vi "test_conv2.vi"() -> ()   [LabVIEW 2018]
uses:
  <vilib>/Analysis/1siggen.llb/Ramp Pattern by Samples.vi
  <vilib>/addons/Modulation/Digital/General/MT Generate Bits (Galois, PN Order).vi
  <vilib>/Analysis/baseanly.llb/Mean (DBL).vi
  <vilib>/addons/Modulation/Analog/support/mod_Set Error Source.vi
  <vilib>/addons/Modulation/Digital/Support/Common/Validators/mod_Generate Bits Validate.vi
  <vilib>/addons/Modulation/Digital/Support/Common/Validators/mod_AWGN Validate.vi
  <vilib>/addons/Modulation/Digital/Impairments/subVIs/mod_createSeeds.vi
  <vilib>/addons/Modulation/Digital/Support/Common/Validators/mod_Validate Samples Per Symbol.vi
  <vilib>/addons/Modulation/Analog/support/Validators/mod_Validate Complex Waveform.vi
  <vilib>/addons/Modulation/Analog/support/Validators/mod_WFErrorHandler.vi
  <vilib>/addons/Modulation/Digital/Support/Common/Validators/mod_Generate Filter Coefficients Validate.vi
  <vilib>/addons/Modulation/Digital/General/subVIs/mod_Generate Filter Coefficients.vi
  <vilib>/addons/Modulation/Digital/General/MT Generate PSK System Parameters(M).vi
  <vilib>/addons/Modulation/Digital/General/subVIs/mod_Generate Bits PN Sequence.vi
  <vilib>/Analysis/1siggen.llb/Gaussian White Noise (obs 90).vi
  <vilib>/addons/Modulation/Digital/General/MT Apply Matched Filter (Generic).vi
  <vilib>/addons/Modulation/Digital/General/MT Map PSK Symbols to Bits.vi
  <vilib>/addons/Modulation/Digital/Channel Coding/MT Convolutional Decoder (Viterbi Hard Decision, Rate).vi
  <vilib>/addons/Modulation/Digital/Demodulation/MT Calculate BER After Trigger (PN Sequence).vi
  <vilib>/addons/Modulation/niDMT.lvlib
  <vilib>/Analysis/NI_AALBase.lvlib
panel:
  out "size(s) 4":i32
  out "bruité":cdb[](array[numeric])
  out "built-in decoder":i8[](array[numeric])
  in  "Traceback Depth (D)":i32=20
  in  "Constraint Length (K)":i32=3
  in  "Rate (k/n)":enum16{"1/2", "1/3", "1/4", "2/3", "3/4"}(ring)
  in  "PN Sequence Order":i32=19
  in  "Seed In":i32=-1
  out "BER vs Eb/N0 (dB)\n[AWGN channel]":cluster{"Ramp Pattern":dbl[], dbl[]}(graph)
  in  "Trials per Eb/N0 Sample":i32=1
  in  "Start Eb/N0 (dB)":dbl=5.0 format="%0.2f"
  in  "End Eb/N0 (dB)":dbl=10.0 format="%0.2f"
  in  "Eb/N0 Samples":i32=6
  out "Progress in current trial":i32(slide) scale=0.0..100.0
  out "Accumulated BER (coding)":dbl format="%.4p"
  out "IQ Constellation":T1(graph)
  out "Y":cdb[](array[numeric])
  out "out_perso":i8[](array[numeric])
  out "size(s)":i32
  out "size(s) 2":i32
  out "message":i8[](array[numeric])
  out "size(s) 3":i32
  out "mess_codé":i8[](array[numeric])
  out "built-in CAN":i8[](array[numeric])
  out "Current trial":i32
  out "Current Eb/N0":dbl
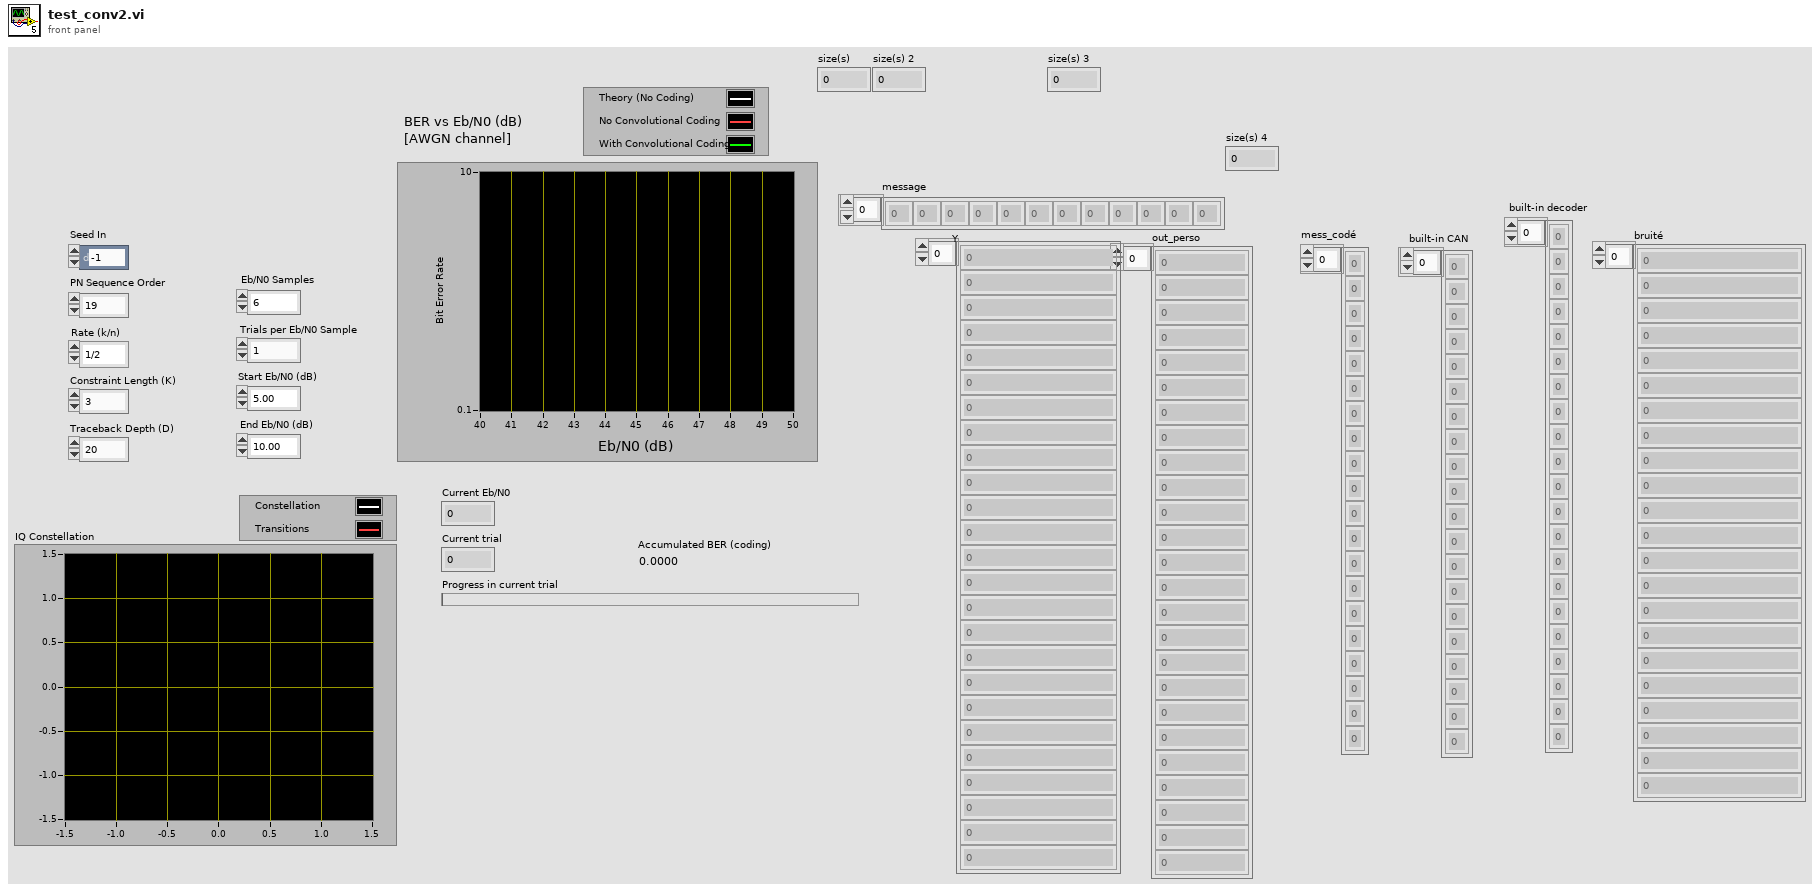
[diagram p1: front panel]
types:
  T1 = cluster{"Decimated Array":dbl[], "Decimated Array":dbl[]}[]
  T2 = enum16{"none", "Raised Cosine", "Root Raised Cos", "Gaussian"}
  T3 = cluster{"samples per symbol (16)":i32, "symbol map":cdb[], "differential PSK":enum16{"disable", "enable"}, "PSK type":u16}
  T4 = typedef "niAMT.lvlib/Complex Data Waveform.ctl" = cluster{"t0":dbl, "dt":dbl, "Y":cdb[]}
  T5 = cluster{"constellation":dbl[], "oversampled data":dbl[]}[]
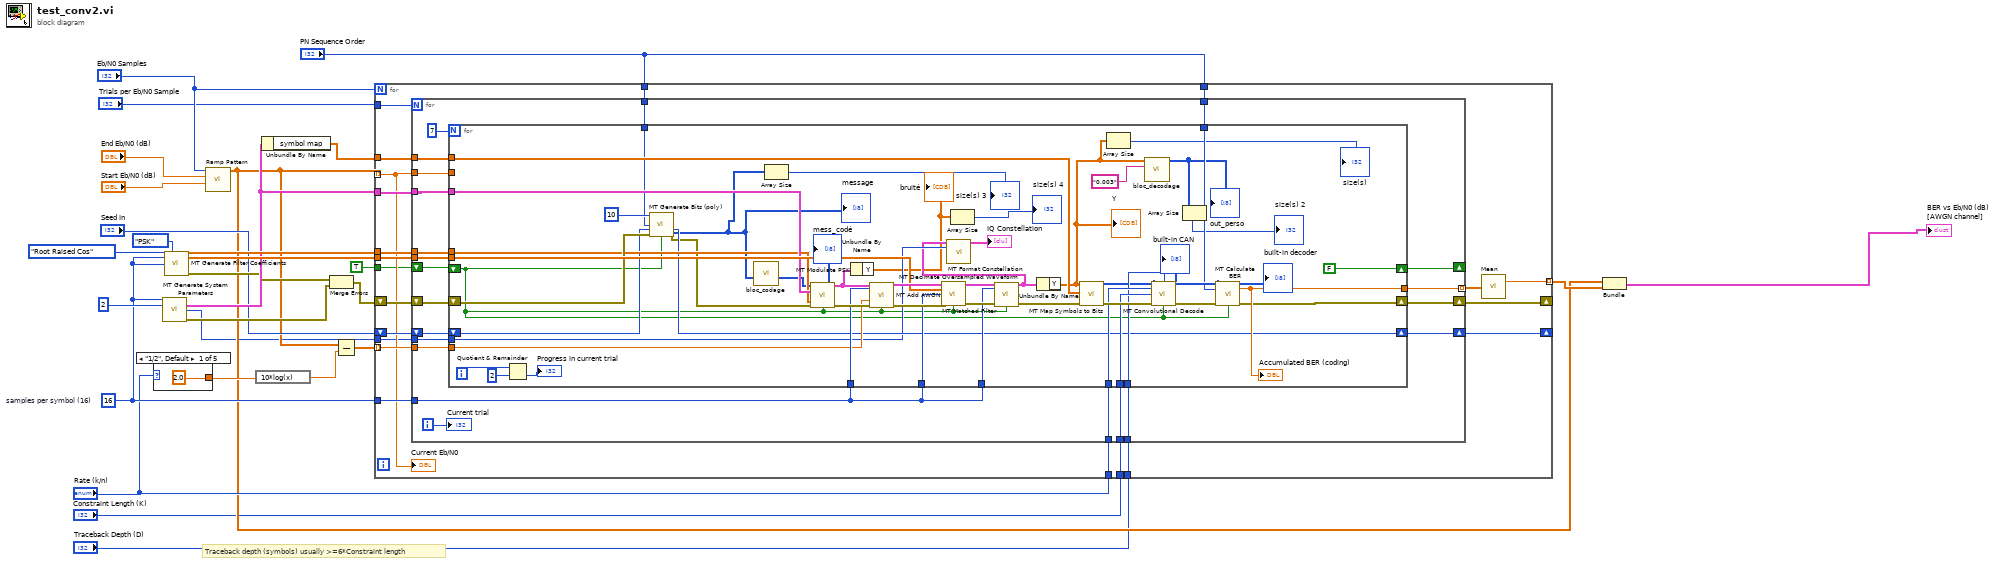
[diagram p0: block diagram]
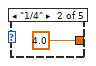
[diagram p2: hidden frame]
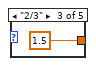
[diagram p3: hidden frame]
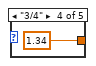
[diagram p4: hidden frame]
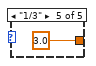
[diagram p5: hidden frame]
diagram:
  w21 = 16  # samples per symbol (16)
  # "Traceback depth (symbols) usually >=6*Constraint length"
  n1 = case shown="\"1/2\", Default" "Rate (k/n)" {
    tunnel: [2.0 4.0 1.5 1.34 3.0] -> w8
    frame "1/2", Default {
    }
    frame "1/4" {
    }
    frame "2/3" {
    }
    frame "3/4" {
    }
    frame "1/3" {
    }
  }
  n2 = call-poly <vilib>:"MT Generate System Parameters.vi"("samples per symbol (16)"=w21, "M-PSK (4)"=2) -> ("PSK system parameters"=w20:T3, "bits per symbol"=w2:i32, "error out"=w15:errorcluster)  [unwired: 11 in]
  n3 = call <vilib>:"MT Generate Filter Coefficients.vi"("pulse shaping filter (none)"=T2."Root Raised Cos", "modulation type"=enum16{"FSK", "PSK", "QAM", "MSK", "PAM", "ASK"}."PSK", "pulse shaping samples per symbol (16)"=w21, "matched samples per symbol (16)"=w21) -> ("pulse shaping filter coefficients"=w26:dbl[], "matched filter coefficients"=w22:dbl[], "error out"=w16:errorcluster)  [unwired: 9 in]
  n4 = call-poly <vilib>:"Ramp Pattern.vi"("start"="Start Eb/N0 (dB)", "end"="End Eb/N0 (dB)", "samples"="Eb/N0 Samples") -> ("Ramp Pattern"=w6:dbl[])  [unwired: 7 in, 1 out]
  n5 = expression code="10*log(x)"(w8) -> (w7:dbl)
  n6 = Unbundle By Name(w20) -> ("symbol map"=w19:cdb[])
  n7 = Merge Errors(w16, w15) -> (w14:errorcluster)
  n8 = Subtract(x=w6, y=w7) -> (x-y=w13:dbl[])
  n9 = for {
    N: "Eb/N0 Samples" -> [_]
    tunnel: w26 -> [w54]
    tunnel: w6 -> [w36] mode=indexing
    tunnel: w22 -> [w52]
    tunnel: w21 -> [w51]
    tunnel: w19 -> [w50]
    tunnel: "Rate (k/n)" -> [w49]
    tunnel: "Constraint Length (K)" -> [w48]
    tunnel: "Traceback Depth (D)" -> [w47]
    tunnel: "Trials per Eb/N0 Sample" -> [w46]
    tunnel: [w44] -> w10 mode=indexing
    tunnel: w20 -> [w53]
    shift-right: [w43] -> _
    shift-left: w14 -> [w42]
    tunnel: w13 -> [w41] mode=indexing
    shift-right: [w39] -> _
    shift-left: "Seed In" -> [w40]
    tunnel: "PN Sequence Order" -> [w38]
    tunnel: "PN Sequence Order" -> [w37]
    tunnel: TRUE ("reset? (T)") -> [w35]
    tunnel: w2 -> [w34]
    n10 = for {
      N: w46 -> [_]
      tunnel: w54 -> [w76]
      tunnel: w36 -> [w74]
      tunnel: w52 -> [w73]
      tunnel: w51 -> [w72]
      tunnel: w50 -> [w71]
      tunnel: w49 -> [w70]
      tunnel: w48 -> [w69]
      tunnel: w47 -> [w68]
      tunnel: [w66] -> w45 mode=indexing
      tunnel: w53 -> [w75]
      shift-right: [w64] -> w43
      shift-left: w42 -> [w63]
      tunnel: w41 -> [w62]
      shift-right: [w60] -> w39
      shift-left: w40 -> [w61]
      tunnel: w38 -> [w59]
      tunnel: w37 -> [w58]
      shift-right: [w56] -> _
      shift-left: w35 -> [w57]
      tunnel: w34 -> [w55]
      i -> [w65]
      n11 = for {
        N: 7 -> [_]
        tunnel: w76 -> [w103]
        shift-right: [FALSE ("reset? (T)")] -> w56
        shift-left: w57 -> [w83]
        tunnel: w74 -> [_]
        tunnel: w73 -> [w122]
        tunnel: w72 -> [w117]
        tunnel: w72 -> [w115]
        tunnel: w72 -> [w116]
        tunnel: w71 -> [w113]
        tunnel: w70 -> [w111]
        tunnel: w69 -> [w110]
        tunnel: w68 -> [w109]
        tunnel: [w105] -> w66
        tunnel: w75 -> [w120]
        shift-right: [w93] -> w64
        shift-left: w63 -> [w104]
        tunnel: w62 -> [w102]
        shift-right: [w100] -> w60
        shift-left: w61 -> [w101]
        tunnel: w59 -> [w99]
        tunnel: w58 -> [w98]
        tunnel: w55 -> [w94]
        i -> [w96]
        n12 = Quotient & Remainder(x=w96, y=2) -> (floor(x/y)=→"Progress in current trial":i32)  [unwired: 1 out]
        n13 = call-poly <vilib>:"MT Generate Bits (poly).vi"("total bits (128)"=10, "PN sequence order (9)"=w99, "seed in (0xD6BF7DF2)"=w101, "error in (no error)"=w104, "reset? (T)"=w83) -> ("output bit stream"=w81:i8[], "seed out"=w100:i32, "error out"=w82:errorcluster)  [unwired: 8 in]
        "message" <- w81
        n14 = call "bloc_codage.vi"("Array in"=w81) -> ("output bit stream"=w80:i8[])  [unwired: 8 in, 2 out]
        "mess_codé" <- w80
        n15 = Array Size(array=w81) -> (size(s)=→"size(s) 3":i32)
        n16 = call <vilib>:"MT Modulate PSK.vi"("input bit stream"=w80, "PSK system parameters"=w120, "pulse shaping filter coefficients"=w103, "error in (no error)"=w82, "reset? (T)"=w83) -> ("output complex waveform"=w79:T4, "error out"=w121:errorcluster)  [unwired: 8 in, 1 out]
        n17 = Unbundle By Name(w79) -> ("Y"=w78:cdb[])
        "bruité" <- w78
        n18 = call <vilib>:"MT Add AWGN.vi"("input complex waveform"=w79, "samples per symbol (16)"=w116, "Eb/N0 (10 dB)"=w102, "error in (no error)"=w121, "reset? (T)"=w83) -> ("output complex waveform"=w123:T4, "error out"=w124:errorcluster)  [unwired: 8 in, 1 out]
        n19 = call-poly <vilib>:"MT Matched Filter.vi"("input complex waveform"=w123, "matched filter coefficients"=w122, "samples per symbol (16)"=w115, "error in (no error)"=w124, "reset? (T)"=w83) -> ("output complex waveform"=w119:T4, "error out"=w118:errorcluster)  [unwired: 9 in]
        n20 = Array Size(array=w78) -> (size(s)=→"size(s) 4":i32)
        n21 = call <vilib>:"MT Decimate Oversampled Waveform.vi"("input complex waveform"=w119, "decimation factor"=w117, "error in (no error)"=w118, "reset? (T)"=w83) -> ("output complex waveform"=w92:T4, "error out"=w114:errorcluster)  [unwired: 10 in]
        n22 = call <vilib>:"MT Format Constellation.vi"("waveform"=w92, "samples per symbol"=w94) -> ("constellation graph"=→"IQ Constellation":T5)  [unwired: 12 in, 1 out]
        n23 = Unbundle By Name(w92) -> ("Y"=w88:cdb[])
        "Y" <- w88
        n24 = call-poly <vilib>:"MT Map Symbols to Bits.vi"("symbols"=w88, "symbol map"=w113, "error in (no error)"=w114) -> ("output bit stream"=w90:i8[], "error out"=w112:errorcluster)  [unwired: 11 in]
        "built-in CAN" <- w90
        n25 = Array Size(array=w88) -> (size(s)=→"size(s)":i32)
        n26 = call "bloc_decodage.vi"("sigma2"="0.003", "Array"=w88) -> ("output bit stream"=w85:i8[])  [unwired: 7 in, 2 out]
        "out_perso" <- w85
        n27 = call-poly <vilib>:"MT Convolutional Decode.vi"("input bit stream"=w90, "traceback depth (D)"=w109, "rate (k/n)"=w111, "constraint length (K)"=w110, "error in (no error)"=w112, "reset? (T)"=w83) -> ("output bit stream"=w107:i8[], "error out"=w108:errorcluster)  [unwired: 7 in, 1 out]
        "built-in decoder" <- w107
        n28 = Array Size(array=w85) -> (size(s)=→"size(s) 2":i32)
        n29 = call-poly <vilib>:"MT Calculate BER.vi"("input bit stream"=w107, "PN sequence order (9)"=w98, "error in (no error)"=w108, "reset? (T)"=w83) -> ("accumulated BER"=w105:dbl, "error out"=w93:errorcluster)  [unwired: 7 in, 3 out]
        "Accumulated BER (coding)" <- w105
      }
      "Current trial" <- w65
    }
    n30 = call-poly <vilib>:"Mean.vi"("X"=w45) -> ("mean"=w44:dbl)  [unwired: 1 out]
    "Current Eb/N0" <- w36
  }
  n31 = Bundle("Ramp Pattern"=w6, w10) -> (→"BER vs Eb/N0 (dB)\n[AWGN channel]":cluster{"Ramp Pattern":dbl[], dbl[]})  [unwired: 1 in]
